vi "Cleanup VI BD.vi"(8 "error in (no error)":errorcluster, 11 "VI in":refnum<vi>) -> (0 "error out":errorcluster, 3 "VI out":refnum<vi>)   [LabVIEW 2019, in "gRPC Scripting Tools.lvlib"]
uses:
  gRPC Scripting Tools.lvlib
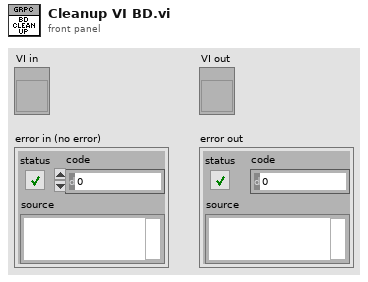
[diagram p1: front panel]
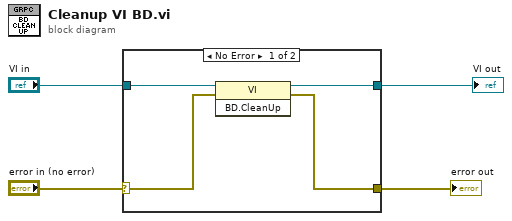
[diagram p0: block diagram]
diagram:
  n1 = case shown="No Error" "error in (no error)" {
    selector: "error in (no error)" -> [w5 w9]
    tunnel: [w8 w9] -> w4
    tunnel: [w7 w10] -> w3
    tunnel: "VI in" -> [w6 w10]
    frame No Error {
      n2 = invoke class="VI" method="BD.CleanUp"(reference=w6, error in=w5) -> (reference out=w7:refnum<vi>, error out=w8:errorcluster)  [unwired: 1 in, 1 out]
    }
    frame Error {
    }
  }
  "error out" <- w4
  "VI out" <- w3
